vi "Autonomous Independent.vi"   [LabVIEW 2020]
doc: "This VI is called when autonomous begins, and will automatically be terminated when autonomous ends. You can carry out timed or sensor driven robot movement independently without needing to return to the caller."
uses:
  <vilib>/Rock Robotics/WPI/Utilities/WPI_GetSetVariantRefNum.vi
  <vilib>/Rock Robotics/Network Tables/NT Read String.vi
  <vilib>/Rock Robotics/Network Tables/NT Write Numeric Array.vi
panel:
  # "Be sure to right-click and choose Data Operations>>Make Current Value default if you want to save the array values with the VI"
  # "Click here to set max"
  # "Click here to set min"
types:
  T1 = typedef "WPI_JoystickDevRef.ctl" = cluster{"Device":T2}
  T2 = typedef "WPI_JoystickDeviceEnum.ctl" = enum16{"USB 0", "USB 1", "USB 2", "USB 3", "USB 4", "USB 5"}
  T3 = typedef "WPI_MotorControlDeviceRef.ctl" = cluster{"DeviceStatus":errorcluster, "Type":T4, "PWM":cluster{"PWM Channel":T5, "DeadBand":T6}, "CAN":cluster{"Device Number":u8, "SetOutput VI Ref":variant, "GetOutput VI Ref":variant, "Enable VI Ref":variant, "Disable VI Ref":variant, "Data":variant}, "Invert":bool, "DIO PWM":cluster{"PWM \"Enable\" Channel":T5, "DIOChannel":T7, "PWM Rate":dbl}}
  T4 = typedef "WPI_MotorControlType.ctl" = enum16{"PWM", "CAN", "DIO PWM"}
  T5 = typedef "FPGA_DIOPWMChannel.ctl" = enum8{"PWM 0", "PWM 1", "PWM 2", "PWM 3", "PWM 4", "PWM 5", "PWM 6", "PWM 7", "PWM 8", "PWM 9", "PWM MXP 0", "PWM MXP 1", "PWM MXP 2", "PWM MXP 3", "PWM MXP 4", "PWM MXP 5", "PWM MXP 6", "PWM MXP 7", "PWM MXP 8", "PWM MXP 9", "Invalid"}
  T6 = typedef "WPI_PWMDeadband.ctl" = cluster{"Name":string, "maxPositivePwm":i32, "minPositivePwm":i32, "centerPwm":i32, "maxNegativePwm":i32, "minNegativePwm":i32, "angularRange":u16}
  T7 = typedef "FPGA_DIOChannel.ctl" = enum8{"DIO 0", "DIO 1", "DIO 2", "DIO 3", "DIO 4", "DIO 5", "DIO 6", "DIO 7", "DIO 8", "DIO 9", "DIO MXP 0", "DIO MXP 1", "DIO MXP 2", "DIO MXP 3", "DIO MXP 4", "DIO MXP 5", "DIO MXP 6", "DIO MXP 7", "DIO MXP 8", "DIO MXP 9", "DIO MXP 10", "DIO MXP 11", "DIO MXP 12", "DIO MXP 13", "DIO MXP 14", "DIO MXP 15", "SPI Port CS1", "SPI Port CS2", "SPI Port CS3", "SPI Port MISO", "SPI Port MOSI", "Invalid"}
  T8 = typedef "WPI_RobotDriveDevRef.ctl" = cluster{"DevStatus":errorcluster, "Motors[]":T3[], "Square Inputs":bool, "Max Output":dbl}
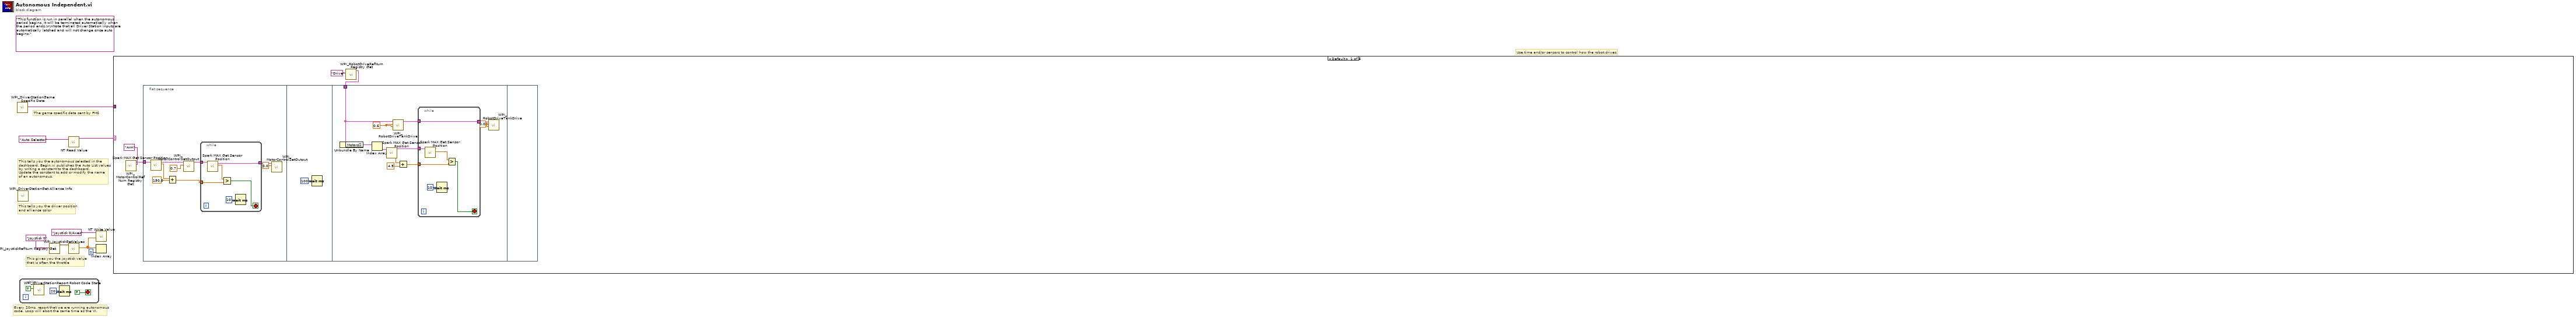
[diagram p0: block diagram]
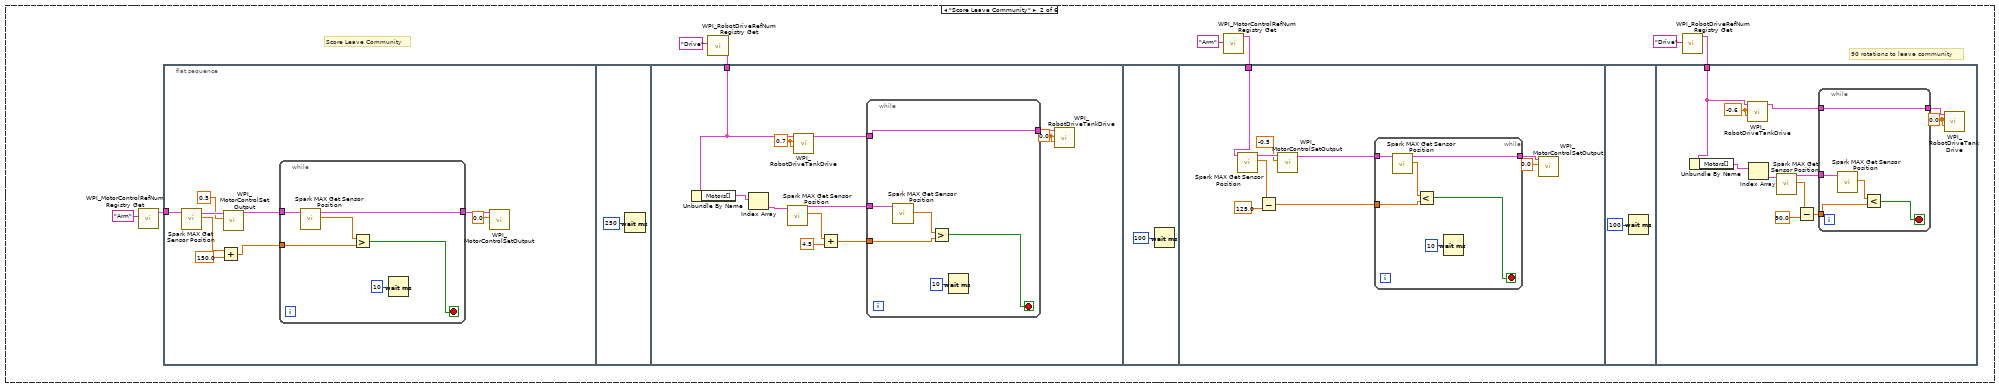
[diagram p2: hidden frame]
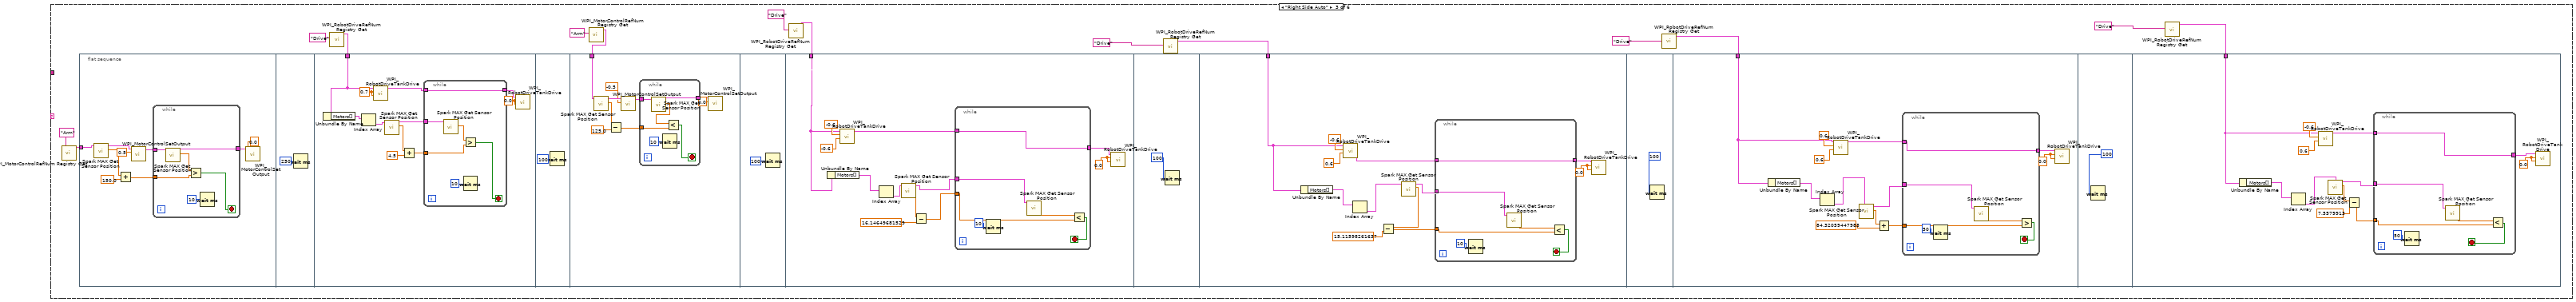
[diagram p3: hidden frame]
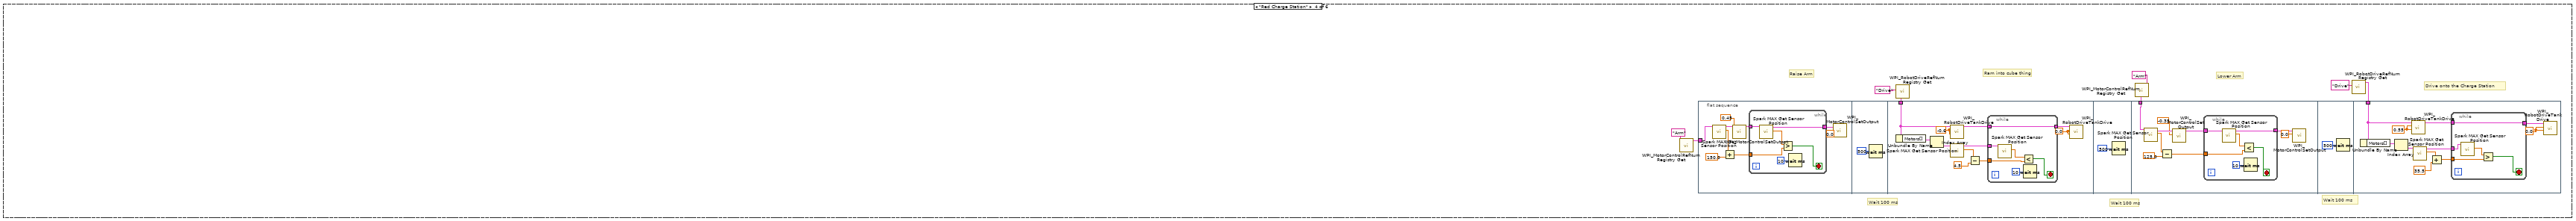
[diagram p4: hidden frame]
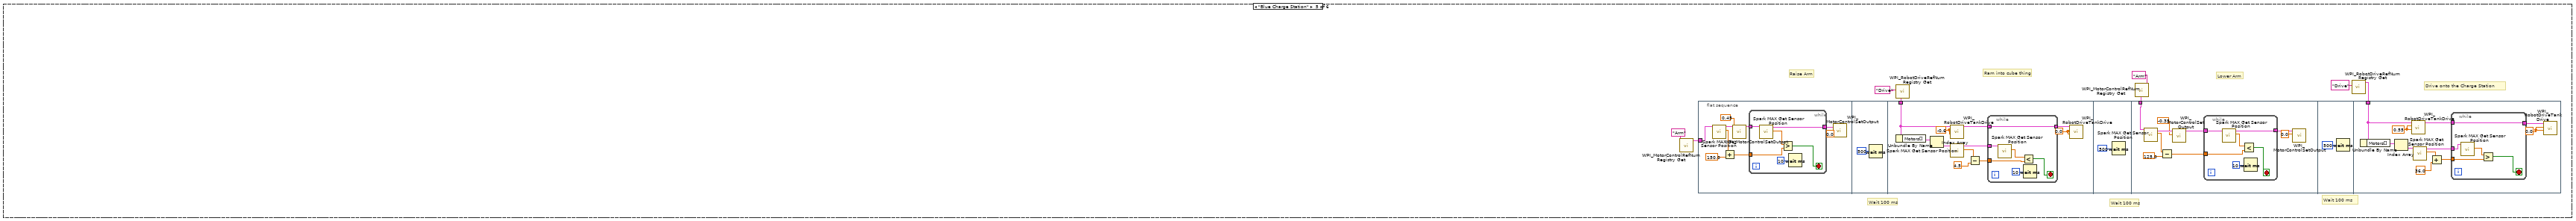
[diagram p5: hidden frame]
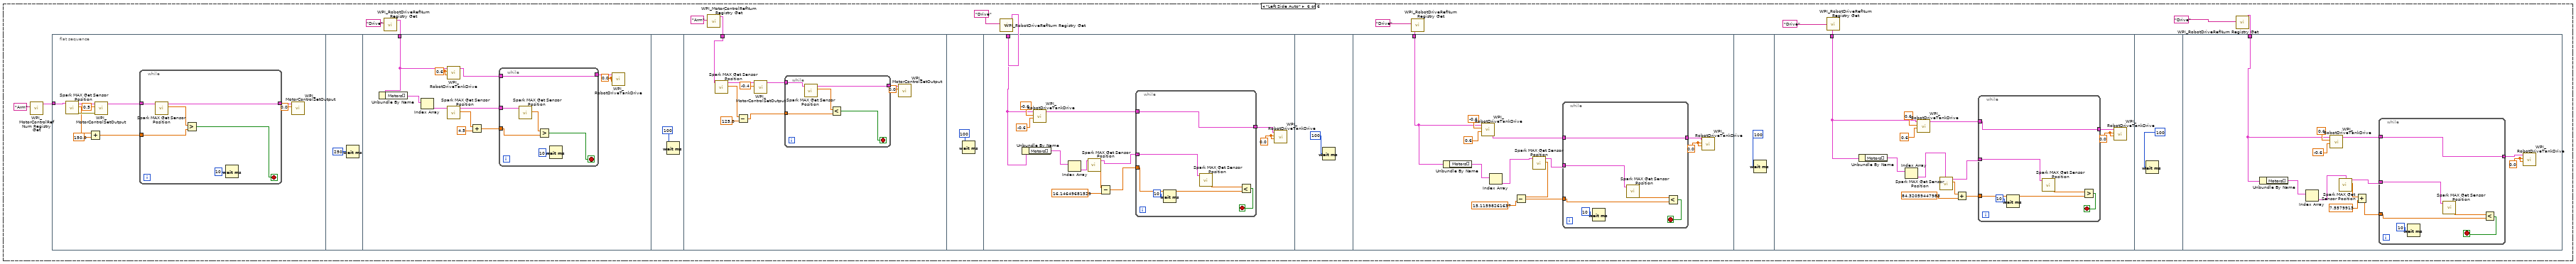
[diagram p6: hidden frame]
diagram:
  (unwired) "This function is run in parallel when the autonomous period begins. It will be terminated automatically when the period ends.\n\nNote that all Driver Station inputs are automatically latched and will not change once auto begins."
  # "The game specific data sent by FMS"
  # "This tells you the autonomous selected in the \ndashboard. Begin.vi publishes the Auto List values\nby writing a constant to the dashboard.\nUpdate the constant to add or modify the name\nof an autonomous."
  # "Every 20ms, report that we are running autonomous\ncode. Loop will abort the same time as the VI."
  # "This gives you the joystick value\nthat is often the throttle"
  # "Use time and/or sensors to control how the robot drives."
  # "This tells you the driver position\nand alliance color"
  n1 = call <vilib>:"WPI_DriverStationGame Specific Data.vi"() -> ("Game Specific Data"=w1:string)  [unwired: 11 in]
  n2 = call <vilib>:"WPI_DriverStationGet Alliance Info.vi"() -> ()  [unwired: 12 out]
  n3 = while {
    stop <- FALSE stop-if-true
    n4 = call <vilib>:"WPI_DriverStationReport Robot Code State.vi"("Autonomous"=TRUE) -> ()  [unwired: 10 in, 1 out]
    n5 = Wait (ms)(milliseconds to wait=u32 20) -> ()  [unwired: 1 out]
  }
  n6 = call <vilib>:"WPI_JoystickRefNum Registry Get.vi"("refnum name"="Joystick 0") -> ("JoystickDevRef"=w7:T1)  [unwired: 1 in, 9 out]
  n7 = call <vilib>:"WPI_JoystickGetValues.vi"("JoystickDevRef"=w7) -> ("Axes"=w3:dbl[])  [unwired: 6 in, 4 out]
  n8 = call-poly <vilib>:"NT Read Value.vi"("name"="Auto Selector" ("Name")) -> ("value"=w4:string)  [unwired: 8 in, 2 out]
  n9 = call-poly <vilib>:"NT Write Value.vi"("value"=w3, "name"="Joystick 0/Axes" ("Name")) -> ()  [unwired: 9 in, 1 out]
  n10 = Index Array(array=w3, index=2) -> ()  [unwired: 1 out]
  n11 = case shown="Default" w4 {
    tunnel: w1 -> [_ _ _ _ _ _]
    frame Default {
      n12 = call <vilib>:"WPI_MotorControlRefNum Registry Get.vi"("refnum name"="Arm") -> ("MotorControlDevRef"=w14:T3)  [unwired: 9 in, 1 out]
      n13 = flat-sequence {
        tunnel: w14 -> [w24]
        tunnel: w12 -> [w41]
        frame #0 {
          n14 = call <vilib>:"Spark MAX Get Sensor Position.vi"("MotorControlDevRef in"=w24) -> ("Sensor Position"=w23:dbl, "MotorControlDevRef out"=w21:T3)  [unwired: 7 in, 2 out]
          n15 = Add(x=w23, y=150.0) -> (x+y=w18:dbl)
          n16 = call <vilib>:"WPI_MotorControlSetOutput.vi"("Output"=0.7, "MotorControlDevRef"=w21) -> ("MotorControlDevRef"=w19:T3)  [unwired: 7 in, 2 out]
          n17 = while {
            tunnel: w19 -> [w30]
            tunnel: w18 -> [w28]
            tunnel: [w25] -> w17
            stop <- w27 stop-if-true
            n18 = call <vilib>:"Spark MAX Get Sensor Position.vi"("MotorControlDevRef in"=w30) -> ("Sensor Position"=w29:dbl, "MotorControlDevRef out"=w25:T3)  [unwired: 7 in, 2 out]
            n19 = Greater?(x=w29, y=w28) -> (0:w27:bool)
            n20 = Wait (ms)(milliseconds to wait=u32 10) -> ()  [unwired: 1 out]
          }
          n21 = call <vilib>:"WPI_MotorControlSetOutput.vi"("Output"=0.0, "MotorControlDevRef"=w17) -> ()  [unwired: 7 in, 3 out]
        }
        frame #1 {
          n22 = Wait (ms)(milliseconds to wait=u32 100) -> ()  [unwired: 1 out]
        }
        frame #2 {
          w32 = 0.0 ("Left axis value")
          w38 = 0.6 ("Left axis value")
          n23 = Unbundle By Name(w41) -> ("Motors[]"=w42:T3[])
          n24 = Index Array(array=w42) -> (element=w40:T3)  [unwired: 1 in]
          n25 = call <vilib>:"Spark MAX Get Sensor Position.vi"("MotorControlDevRef in"=w40) -> ("Sensor Position"=w39:dbl, "MotorControlDevRef out"=w36:T3)  [unwired: 7 in, 2 out]
          n26 = call <vilib>:"WPI_RobotDriveTankDrive.vi"("Right axis value"=w38, "Left axis value"=w38, "RobotDriveDevRef"=w41) -> ("RobotDriveDevRef"=w34:T8)  [unwired: 6 in, 2 out]
          n27 = Add(x=w39, y=4.5) -> (x+y=w35:dbl)
          n28 = while {
            tunnel: w36 -> [w48]
            tunnel: w35 -> [w47]
            tunnel: [w43] -> w33
            tunnel: w34 -> [w43]
            stop <- w45 stop-if-true
            n29 = call <vilib>:"Spark MAX Get Sensor Position.vi"("MotorControlDevRef in"=w48) -> ("Sensor Position"=w46:dbl)  [unwired: 7 in, 3 out]
            n30 = Wait (ms)(milliseconds to wait=u32 10) -> ()  [unwired: 1 out]
            n31 = Greater?(x=w46, y=w47) -> (0:w45:bool)
          }
          n32 = call <vilib>:"WPI_RobotDriveTankDrive.vi"("Right axis value"=w32, "Left axis value"=w32, "RobotDriveDevRef"=w33) -> ()  [unwired: 6 in, 3 out]
        }
        frame #3 {
        }
      }
      n33 = call <vilib>:"WPI_RobotDriveRefNum Registry Get.vi"("refnum name"="Drive") -> ("RobotDriveDevRef"=w12:T8)  [unwired: 9 in, 1 out]
    }
    frame "Score Leave Community" {
      # "90 rotations to leave community"
      # "Score Leave Community"
      n34 = call <vilib>:"WPI_MotorControlRefNum Registry Get.vi"("refnum name"="Arm") -> ("MotorControlDevRef"=w55:T3)  [unwired: 9 in, 1 out]
      n35 = flat-sequence {
        tunnel: w55 -> [w65]
        tunnel: w53 -> [w82]
        tunnel: w51 -> [w99]
        tunnel: w49 -> [w115]
        frame #0 {
          n36 = call <vilib>:"Spark MAX Get Sensor Position.vi"("MotorControlDevRef in"=w65) -> ("Sensor Position"=w63:dbl, "MotorControlDevRef out"=w64:T3)  [unwired: 7 in, 2 out]
          n37 = Add(x=w63, y=150.0) -> (x+y=w59:dbl)
          n38 = call <vilib>:"WPI_MotorControlSetOutput.vi"("Output"=0.5, "MotorControlDevRef"=w64) -> ("MotorControlDevRef"=w60:T3)  [unwired: 7 in, 2 out]
          n39 = while {
            tunnel: w60 -> [w71]
            tunnel: w59 -> [w69]
            tunnel: [w66] -> w58
            stop <- w68 stop-if-true
            n40 = call <vilib>:"Spark MAX Get Sensor Position.vi"("MotorControlDevRef in"=w71) -> ("Sensor Position"=w70:dbl, "MotorControlDevRef out"=w66:T3)  [unwired: 7 in, 2 out]
            n41 = Greater?(x=w70, y=w69) -> (0:w68:bool)
            n42 = Wait (ms)(milliseconds to wait=u32 10) -> ()  [unwired: 1 out]
          }
          n43 = call <vilib>:"WPI_MotorControlSetOutput.vi"("Output"=0.0, "MotorControlDevRef"=w58) -> ()  [unwired: 7 in, 3 out]
        }
        frame #1 {
          n44 = Wait (ms)(milliseconds to wait=u32 250) -> ()  [unwired: 1 out]
        }
        frame #2 {
          w73 = 0.0 ("Left axis value")
          w78 = 0.7 ("Left axis value")
          n45 = Unbundle By Name(w82) -> ("Motors[]"=w83:T3[])
          n46 = Index Array(array=w83) -> (element=w81:T3)  [unwired: 1 in]
          n47 = call <vilib>:"Spark MAX Get Sensor Position.vi"("MotorControlDevRef in"=w81) -> ("Sensor Position"=w80:dbl, "MotorControlDevRef out"=w77:T3)  [unwired: 7 in, 2 out]
          n48 = call <vilib>:"WPI_RobotDriveTankDrive.vi"("Right axis value"=w78, "Left axis value"=w78, "RobotDriveDevRef"=w82) -> ("RobotDriveDevRef"=w75:T8)  [unwired: 6 in, 2 out]
          n49 = Add(x=w80, y=4.5) -> (x+y=w76:dbl)
          n50 = while {
            tunnel: w77 -> [w89]
            tunnel: w76 -> [w87]
            tunnel: w75 -> [w84]
            tunnel: [w84] -> w74
            stop <- w86 stop-if-true
            n51 = call <vilib>:"Spark MAX Get Sensor Position.vi"("MotorControlDevRef in"=w89) -> ("Sensor Position"=w88:dbl)  [unwired: 7 in, 3 out]
            n52 = Greater?(x=w88, y=w87) -> (0:w86:bool)
            n53 = Wait (ms)(milliseconds to wait=u32 10) -> ()  [unwired: 1 out]
          }
          n54 = call <vilib>:"WPI_RobotDriveTankDrive.vi"("Right axis value"=w73, "Left axis value"=w73, "RobotDriveDevRef"=w74) -> ()  [unwired: 6 in, 3 out]
        }
        frame #3 {
          n55 = Wait (ms)(milliseconds to wait=u32 100) -> ()  [unwired: 1 out]
        }
        frame #4 {
          n56 = call <vilib>:"Spark MAX Get Sensor Position.vi"("MotorControlDevRef in"=w99) -> ("Sensor Position"=w96:dbl, "MotorControlDevRef out"=w98:T3)  [unwired: 7 in, 2 out]
          n57 = Subtract(x=w96, y=125.0) -> (x-y=w93:dbl)
          n58 = call <vilib>:"WPI_MotorControlSetOutput.vi"("Output"=-0.5, "MotorControlDevRef"=w98) -> ("MotorControlDevRef"=w94:T3)  [unwired: 7 in, 2 out]
          n59 = while {
            tunnel: w94 -> [w105]
            tunnel: w93 -> [w103]
            tunnel: [w100] -> w92
            stop <- w102 stop-if-true
            n60 = call <vilib>:"Spark MAX Get Sensor Position.vi"("MotorControlDevRef in"=w105) -> ("Sensor Position"=w104:dbl, "MotorControlDevRef out"=w100:T3)  [unwired: 7 in, 2 out]
            n61 = Less?(x=w104, y=w103) -> (x < y?=w102:bool)
            n62 = Wait (ms)(milliseconds to wait=u32 10) -> ()  [unwired: 1 out]
          }
          n63 = call <vilib>:"WPI_MotorControlSetOutput.vi"("Output"=0.0, "MotorControlDevRef"=w92) -> ()  [unwired: 7 in, 3 out]
        }
        frame #5 {
          n64 = Wait (ms)(milliseconds to wait=u32 100) -> ()  [unwired: 1 out]
        }
        frame #6 {
          w109 = 0.0 ("Left axis value")
          w116 = -0.6 ("Left axis value")
          n65 = Unbundle By Name(w115) -> ("Motors[]"=w117:T3[])
          n66 = call <vilib>:"WPI_RobotDriveTankDrive.vi"("Right axis value"=w116, "Left axis value"=w116, "RobotDriveDevRef"=w115) -> ("RobotDriveDevRef"=w108:T8)  [unwired: 6 in, 2 out]
          n67 = Index Array(array=w117) -> (element=w114:T3)  [unwired: 1 in]
          n68 = call <vilib>:"Spark MAX Get Sensor Position.vi"("MotorControlDevRef in"=w114) -> ("Sensor Position"=w113:dbl, "MotorControlDevRef out"=w111:T3)  [unwired: 7 in, 2 out]
          n69 = Subtract(x=w113, y=90.0) -> (x-y=w110:dbl)
          n70 = while {
            tunnel: w111 -> [w122]
            tunnel: w110 -> [w121]
            tunnel: [w118] -> w107
            tunnel: w108 -> [w118]
            stop <- w119 stop-if-true
            n71 = call <vilib>:"Spark MAX Get Sensor Position.vi"("MotorControlDevRef in"=w122) -> ("Sensor Position"=w120:dbl)  [unwired: 7 in, 3 out]
            n72 = Less?(x=w120, y=w121) -> (x < y?=w119:bool)
          }
          n73 = call <vilib>:"WPI_RobotDriveTankDrive.vi"("Right axis value"=w109, "Left axis value"=w109, "RobotDriveDevRef"=w107) -> ()  [unwired: 6 in, 3 out]
        }
      }
      n74 = call <vilib>:"WPI_RobotDriveRefNum Registry Get.vi"("refnum name"="Drive") -> ("RobotDriveDevRef"=w53:T8)  [unwired: 9 in, 1 out]
      n75 = call <vilib>:"WPI_MotorControlRefNum Registry Get.vi"("refnum name"="Arm") -> ("MotorControlDevRef"=w51:T3)  [unwired: 9 in, 1 out]
      n76 = call <vilib>:"WPI_RobotDriveRefNum Registry Get.vi"("refnum name"="Drive") -> ("RobotDriveDevRef"=w49:T8)  [unwired: 9 in, 1 out]
    }
    frame "Right Side Auto" {
      n77 = call <vilib>:"WPI_MotorControlRefNum Registry Get.vi"("refnum name"="Arm") -> ("MotorControlDevRef"=w127:T3)  [unwired: 9 in, 1 out]
      n78 = flat-sequence {
        tunnel: w127 -> [w145]
        tunnel: w125 -> [w162]
        tunnel: w123 -> [w179]
        tunnel: w135 -> [w193]
        tunnel: w133 -> [w210]
        tunnel: w131 -> [w227]
        tunnel: w129 -> [w244]
        frame #0 {
          n79 = call <vilib>:"Spark MAX Get Sensor Position.vi"("MotorControlDevRef in"=w145) -> ("Sensor Position"=w144:dbl, "MotorControlDevRef out"=w142:T3)  [unwired: 7 in, 2 out]
          n80 = Add(x=w144, y=150.0) -> (x+y=w137:dbl)
          n81 = call <vilib>:"WPI_MotorControlSetOutput.vi"("Output"=0.5, "MotorControlDevRef"=w142) -> ("MotorControlDevRef"=w140:T3)  [unwired: 7 in, 2 out]
          n82 = while {
            tunnel: w140 -> [w151]
            tunnel: [w150] -> w139
            tunnel: w137 -> [w148]
            stop <- w147 stop-if-true
            n83 = call <vilib>:"Spark MAX Get Sensor Position.vi"("MotorControlDevRef in"=w151) -> ("Sensor Position"=w149:dbl, "MotorControlDevRef out"=w150:T3)  [unwired: 7 in, 2 out]
            n84 = Greater?(x=w149, y=w148) -> (0:w147:bool)
            n85 = Wait (ms)(milliseconds to wait=u32 10) -> ()  [unwired: 1 out]
          }
          n86 = call <vilib>:"WPI_MotorControlSetOutput.vi"("Output"=0.0, "MotorControlDevRef"=w139) -> ()  [unwired: 7 in, 3 out]
        }
        frame #1 {
          n87 = Wait (ms)(milliseconds to wait=u32 250) -> ()  [unwired: 1 out]
        }
        frame #2 {
          w154 = 0.7 ("Left axis value")
          w153 = 0.0 ("Left axis value")
          n88 = Unbundle By Name(w162) -> ("Motors[]"=w163:T3[])
          n89 = Index Array(array=w163) -> (element=w161:T3)  [unwired: 1 in]
          n90 = call <vilib>:"WPI_RobotDriveTankDrive.vi"("Right axis value"=w154, "Left axis value"=w154, "RobotDriveDevRef"=w162) -> ("RobotDriveDevRef"=w155:T8)  [unwired: 6 in, 2 out]
          n91 = call <vilib>:"Spark MAX Get Sensor Position.vi"("MotorControlDevRef in"=w161) -> ("Sensor Position"=w159:dbl, "MotorControlDevRef out"=w158:T3)  [unwired: 7 in, 2 out]
          n92 = Add(x=w159, y=4.5) -> (x+y=w157:dbl)
          n93 = while {
            tunnel: w158 -> [w169]
            tunnel: w157 -> [w167]
            tunnel: w155 -> [w164]
            tunnel: [w164] -> w156
            stop <- w166 stop-if-true
            n94 = call <vilib>:"Spark MAX Get Sensor Position.vi"("MotorControlDevRef in"=w169) -> ("Sensor Position"=w168:dbl)  [unwired: 7 in, 3 out]
            n95 = Greater?(x=w168, y=w167) -> (0:w166:bool)
            n96 = Wait (ms)(milliseconds to wait=u32 10) -> ()  [unwired: 1 out]
          }
          n97 = call <vilib>:"WPI_RobotDriveTankDrive.vi"("Right axis value"=w153, "Left axis value"=w153, "RobotDriveDevRef"=w156) -> ()  [unwired: 6 in, 3 out]
        }
        frame #3 {
          n98 = Wait (ms)(milliseconds to wait=u32 100) -> ()  [unwired: 1 out]
        }
        frame #4 {
          n99 = call <vilib>:"Spark MAX Get Sensor Position.vi"("MotorControlDevRef in"=w179) -> ("Sensor Position"=w177:dbl, "MotorControlDevRef out"=w176:T3)  [unwired: 7 in, 2 out]
          n100 = Subtract(x=w177, y=125.0) -> (x-y=w173:dbl)
          n101 = call <vilib>:"WPI_MotorControlSetOutput.vi"("Output"=-0.5, "MotorControlDevRef"=w176) -> ("MotorControlDevRef"=w174:T3)  [unwired: 7 in, 2 out]
          n102 = while {
            tunnel: w174 -> [w185]
            tunnel: w173 -> [w184]
            tunnel: [w180] -> w172
            stop <- w182 stop-if-true
            n103 = call <vilib>:"Spark MAX Get Sensor Position.vi"("MotorControlDevRef in"=w185) -> ("Sensor Position"=w183:dbl, "MotorControlDevRef out"=w180:T3)  [unwired: 7 in, 2 out]
            n104 = Wait (ms)(milliseconds to wait=u32 10) -> ()  [unwired: 1 out]
            n105 = Less?(x=w183, y=w184) -> (x < y?=w182:bool)
          }
          n106 = call <vilib>:"WPI_MotorControlSetOutput.vi"("Output"=0.0, "MotorControlDevRef"=w172) -> ()  [unwired: 7 in, 3 out]
        }
        frame #5 {
          n107 = Wait (ms)(milliseconds to wait=u32 100) -> ()  [unwired: 1 out]
        }
        frame #6 {
          w196 = 0.0
          n108 = Unbundle By Name(w193) -> ("Motors[]"=w198:T3[])
          n109 = call <vilib>:"WPI_RobotDriveTankDrive.vi"("Right axis value"=-0.6, "Left axis value"=-0.6, "RobotDriveDevRef"=w193) -> ("RobotDriveDevRef"=w192:T8)  [unwired: 6 in, 2 out]
          n110 = Index Array(array=w198) -> (element=w191:T3)  [unwired: 1 in]
          n111 = call <vilib>:"Spark MAX Get Sensor Position.vi"("MotorControlDevRef in"=w191) -> ("Sensor Position"=w189:dbl, "MotorControlDevRef out"=w190:T3)  [unwired: 7 in, 2 out]
          n112 = Subtract(x=w189, y=16.14649681529) -> (x-y=w188:dbl)
          n113 = while {
            tunnel: w190 -> [w202]
            tunnel: [w200] -> w197
            tunnel: w192 -> [w200]
            tunnel: w188 -> [w199]
            stop <- w203 stop-if-true
            n114 = Wait (ms)(milliseconds to wait=10) -> ()  [unwired: 1 out]
            n115 = call <vilib>:"Spark MAX Get Sensor Position.vi"("MotorControlDevRef in"=w202) -> ("Sensor Position"=w204:dbl)  [unwired: 7 in, 3 out]
            n116 = Less?(x=w204, y=w199) -> (x < y?=w203:bool)
          }
          n117 = call <vilib>:"WPI_RobotDriveTankDrive.vi"("Right axis value"=w196, "Left axis value"=w196, "RobotDriveDevRef"=w197) -> ()  [unwired: 6 in, 3 out]
        }
        frame #7 {
          n118 = Wait (ms)(milliseconds to wait=100) -> ()  [unwired: 1 out]
        }
        frame #8 {
          w214 = 0.0
          n119 = Unbundle By Name(w210) -> ("Motors[]"=w215:T3[])
          n120 = call <vilib>:"WPI_RobotDriveTankDrive.vi"("Right axis value"=0.6, "Left axis value"=-0.6, "RobotDriveDevRef"=w210) -> ("RobotDriveDevRef"=w209:T8)  [unwired: 6 in, 2 out]
          n121 = Index Array(array=w215) -> (element=w217:T3)  [unwired: 1 in]
          n122 = call <vilib>:"Spark MAX Get Sensor Position.vi"("MotorControlDevRef in"=w217) -> ("Sensor Position"=w208:dbl, "MotorControlDevRef out"=w216:T3)  [unwired: 7 in, 2 out]
          n123 = Subtract(x=w208, y=15.11598261637) -> (x-y=w206:dbl)
          n124 = while {
            tunnel: w216 -> [w221]
            tunnel: [w219] -> w213
            tunnel: w209 -> [w219]
            tunnel: w206 -> [w218]
            stop <- w222 stop-if-true
            n125 = Wait (ms)(milliseconds to wait=10) -> ()  [unwired: 1 out]
            n126 = call <vilib>:"Spark MAX Get Sensor Position.vi"("MotorControlDevRef in"=w221) -> ("Sensor Position"=w223:dbl)  [unwired: 7 in, 3 out]
            n127 = Less?(x=w223, y=w218) -> (x < y?=w222:bool)
          }
          n128 = call <vilib>:"WPI_RobotDriveTankDrive.vi"("Right axis value"=w214, "Left axis value"=w214, "RobotDriveDevRef"=w213) -> ()  [unwired: 6 in, 3 out]
        }
        frame #9 {
          n129 = Wait (ms)(milliseconds to wait=100) -> ()  [unwired: 1 out]
        }
        frame #10 {
          w233 = 0.0
          n130 = Unbundle By Name(w227) -> ("Motors[]"=w234:T3[])
          n131 = Index Array(array=w234) -> (element=w236:T3)  [unwired: 1 in]
          n132 = call <vilib>:"WPI_RobotDriveTankDrive.vi"("Right axis value"=0.6, "Left axis value"=0.6, "RobotDriveDevRef"=w227) -> ("RobotDriveDevRef"=w226:T8)  [unwired: 6 in, 2 out]
          n133 = call <vilib>:"Spark MAX Get Sensor Position.vi"("MotorControlDevRef in"=w236) -> ("Sensor Position"=w231:dbl, "MotorControlDevRef out"=w235:T3)  [unwired: 7 in, 2 out]
          n134 = Add(x=w231, y=84.32059447983 ("Position")) -> (x+y=w225:dbl)
          n135 = while {
            tunnel: w235 -> [w240]
            tunnel: [w238] -> w232
            tunnel: w226 -> [w238]
            tunnel: w225 -> [w237]
            stop <- w241 stop-if-true
            n136 = Wait (ms)(milliseconds to wait=50) -> ()  [unwired: 1 out]
            n137 = call <vilib>:"Spark MAX Get Sensor Position.vi"("MotorControlDevRef in"=w240) -> ("Sensor Position"=w242:dbl)  [unwired: 7 in, 3 out]
            n138 = Greater?(x=w242, y=w237) -> (0:w241:bool)
          }
          n139 = call <vilib>:"WPI_RobotDriveTankDrive.vi"("Right axis value"=w233, "Left axis value"=w233, "RobotDriveDevRef"=w232) -> ()  [unwired: 6 in, 3 out]
        }
        frame #11 {
          n140 = Wait (ms)(milliseconds to wait=100) -> ()  [unwired: 1 out]
        }
        frame #12 {
          w252 = 0.0
          n141 = Unbundle By Name(w244) -> ("Motors[]"=w253:T3[])
          n142 = Index Array(array=w253) -> (element=w255:T3)  [unwired: 1 in]
          n143 = call <vilib>:"WPI_RobotDriveTankDrive.vi"("Right axis value"=0.6, "Left axis value"=-0.6, "RobotDriveDevRef"=w244) -> ("RobotDriveDevRef"=w245:T8)  [unwired: 6 in, 2 out]
          n144 = call <vilib>:"Spark MAX Get Sensor Position.vi"("MotorControlDevRef in"=w255) -> ("Sensor Position"=w250:dbl, "MotorControlDevRef out"=w254:T3)  [unwired: 7 in, 2 out]
          n145 = Subtract(x=w250, y=7.5579913 ("Position")) -> (x-y=w248:dbl)
          n146 = while {
            tunnel: w254 -> [w259]
            tunnel: [w256] -> w251
            tunnel: w248 -> [w257]
            tunnel: w245 -> [w256]
            stop <- w260 stop-if-true
            n147 = Wait (ms)(milliseconds to wait=50) -> ()  [unwired: 1 out]
            n148 = call <vilib>:"Spark MAX Get Sensor Position.vi"("MotorControlDevRef in"=w259) -> ("Sensor Position"=w261:dbl)  [unwired: 7 in, 3 out]
            n149 = Less?(x=w261, y=w257) -> (x < y?=w260:bool)
          }
          n150 = call <vilib>:"WPI_RobotDriveTankDrive.vi"("Right axis value"=w252, "Left axis value"=w252, "RobotDriveDevRef"=w251) -> ()  [unwired: 6 in, 3 out]
        }
      }
      n151 = call <vilib>:"WPI_RobotDriveRefNum Registry Get.vi"("refnum name"="Drive") -> ("RobotDriveDevRef"=w125:T8)  [unwired: 9 in, 1 out]
      n152 = call <vilib>:"WPI_MotorControlRefNum Registry Get.vi"("refnum name"="Arm") -> ("MotorControlDevRef"=w123:T3)  [unwired: 9 in, 1 out]
      n153 = call <vilib>:"WPI_RobotDriveRefNum Registry Get.vi"("refnum name"="Drive") -> ("RobotDriveDevRef"=w135:T8)  [unwired: 9 in, 1 out]
      n154 = call <vilib>:"WPI_RobotDriveRefNum Registry Get.vi"("refnum name"="Drive") -> ("RobotDriveDevRef"=w133:T8)  [unwired: 9 in, 1 out]
      n155 = call <vilib>:"WPI_RobotDriveRefNum Registry Get.vi"("refnum name"="Drive") -> ("RobotDriveDevRef"=w131:T8)  [unwired: 9 in, 1 out]
      n156 = call <vilib>:"WPI_RobotDriveRefNum Registry Get.vi"("refnum name"="Drive") -> ("RobotDriveDevRef"=w129:T8)  [unwired: 9 in, 1 out]
    }
    frame "Red Charge Station" {
      # "Wait 100 ms"
      # "Drive onto the Charge Station"
      # "Wait 100 ms"
      # "Wait 100 ms"
      # "Lower Arm"
      # "Ram into cube thing"
      # "Raise Arm"
      n157 = call <vilib>:"WPI_MotorControlRefNum Registry Get.vi"("refnum name"="Arm") -> ("MotorControlDevRef"=w268:T3)  [unwired: 9 in, 1 out]
      n158 = flat-sequence {
        tunnel: w268 -> [w277]
        tunnel: w266 -> [w296]
        tunnel: w264 -> [w312]
        tunnel: w263 -> [w330]
        frame #0 {
          n159 = call <vilib>:"Spark MAX Get Sensor Position.vi"("MotorControlDevRef in"=w277) -> ("Sensor Position"=w273:dbl, "MotorControlDevRef out"=w275:T3)  [unwired: 7 in, 2 out]
          n160 = Add(x=w273, y=150.0) -> (x+y=w270:dbl)
          n161 = call <vilib>:"WPI_MotorControlSetOutput.vi"("Output"=0.45, "MotorControlDevRef"=w275) -> ("MotorControlDevRef"=w276:T3)  [unwired: 7 in, 2 out]
          n162 = while {
            tunnel: w276 -> [w284]
            tunnel: [w282] -> w271
            tunnel: w270 -> [w279]
            stop <- w281 stop-if-true
            n163 = call <vilib>:"Spark MAX Get Sensor Position.vi"("MotorControlDevRef in"=w284) -> ("Sensor Position"=w280:dbl, "MotorControlDevRef out"=w282:T3)  [unwired: 7 in, 2 out]
            n164 = Greater?(x=w280, y=w279) -> (0:w281:bool)
            n165 = Wait (ms)(milliseconds to wait=u32 10) -> ()  [unwired: 1 out]
          }
          n166 = call <vilib>:"WPI_MotorControlSetOutput.vi"("Output"=0.0, "MotorControlDevRef"=w271) -> ()  [unwired: 7 in, 3 out]
        }
        frame #1 {
          n167 = Wait (ms)(milliseconds to wait=u32 500) -> ()  [unwired: 1 out]
        }
        frame #2 {
          w286 = -0.6 ("Left axis value")
          w287 = 0.0 ("Left axis value")
          n168 = Unbundle By Name(w296) -> ("Motors[]"=w295:T3[])
          n169 = Index Array(array=w295) -> (element=w294:T3)  [unwired: 1 in]
          n170 = call <vilib>:"WPI_RobotDriveTankDrive.vi"("Right axis value"=w286, "Left axis value"=w286, "RobotDriveDevRef"=w296) -> ("RobotDriveDevRef"=w291:T8)  [unwired: 6 in, 2 out]
          n171 = call <vilib>:"Spark MAX Get Sensor Position.vi"("MotorControlDevRef in"=w294) -> ("Sensor Position"=w293:dbl, "MotorControlDevRef out"=w290:T3)  [unwired: 7 in, 2 out]
          n172 = Subtract(x=w293, y=4.5) -> (x-y=w289:dbl)
          n173 = while {
            tunnel: [w302] -> w288
            tunnel: w291 -> [w302]
            tunnel: w290 -> [w301]
            tunnel: w289 -> [w300]
            stop <- w298 stop-if-true
            n174 = call <vilib>:"Spark MAX Get Sensor Position.vi"("MotorControlDevRef in"=w301) -> ("Sensor Position"=w299:dbl)  [unwired: 7 in, 3 out]
            n175 = Less?(x=w299, y=w300) -> (x < y?=w298:bool)
            n176 = Wait (ms)(milliseconds to wait=u32 10) -> ()  [unwired: 1 out]
          }
          n177 = call <vilib>:"WPI_RobotDriveTankDrive.vi"("Right axis value"=w287, "Left axis value"=w287, "RobotDriveDevRef"=w288) -> ()  [unwired: 6 in, 3 out]
        }
        frame #3 {
          n178 = Wait (ms)(milliseconds to wait=u32 500) -> ()  [unwired: 1 out]
        }
        frame #4 {
          n179 = call <vilib>:"Spark MAX Get Sensor Position.vi"("MotorControlDevRef in"=w312) -> ("Sensor Position"=w309:dbl, "MotorControlDevRef out"=w311:T3)  [unwired: 7 in, 2 out]
          n180 = Subtract(x=w309, y=125.0) -> (x-y=w307:dbl)
          n181 = call <vilib>:"WPI_MotorControlSetOutput.vi"("Output"=-0.35, "MotorControlDevRef"=w311) -> ("MotorControlDevRef"=w306:T3)  [unwired: 7 in, 2 out]
          n182 = while {
            tunnel: w307 -> [w317]
            tunnel: w306 -> [w315]
            tunnel: [w313] -> w305
            stop <- w314 stop-if-true
            n183 = call <vilib>:"Spark MAX Get Sensor Position.vi"("MotorControlDevRef in"=w315) -> ("Sensor Position"=w316:dbl, "MotorControlDevRef out"=w313:T3)  [unwired: 7 in, 2 out]
            n184 = Less?(x=w316, y=w317) -> (x < y?=w314:bool)
            n185 = Wait (ms)(milliseconds to wait=u32 10) -> ()  [unwired: 1 out]
          }
          n186 = call <vilib>:"WPI_MotorControlSetOutput.vi"("Output"=0.0, "MotorControlDevRef"=w305) -> ()  [unwired: 7 in, 3 out]
        }
        frame #5 {
          n187 = Wait (ms)(milliseconds to wait=u32 500) -> ()  [unwired: 1 out]
        }
        frame #6 {
          w322 = 0.0 ("Right axis value")
          w328 = 0.55 ("Left axis value")
          n188 = Unbundle By Name(w330) -> ("Motors[]"=w329:T3[])
          n189 = Index Array(array=w329) -> (element=w327:T3)  [unwired: 1 in]
          n190 = call <vilib>:"WPI_RobotDriveTankDrive.vi"("Right axis value"=w328, "Left axis value"=w328, "RobotDriveDevRef"=w330) -> ("RobotDriveDevRef"=w321:T8)  [unwired: 6 in, 2 out]
          n191 = call <vilib>:"Spark MAX Get Sensor Position.vi"("MotorControlDevRef in"=w327) -> ("Sensor Position"=w326:dbl, "MotorControlDevRef out"=w324:T3)  [unwired: 7 in, 2 out]
          n192 = Add(x=w326, y=35.5) -> (x+y=w323:dbl)
          n193 = while {
            tunnel: w324 -> [w335]
            tunnel: w323 -> [w334]
            tunnel: [w331] -> w320
            tunnel: w321 -> [w331]
            stop <- w332 stop-if-true
            n194 = call <vilib>:"Spark MAX Get Sensor Position.vi"("MotorControlDevRef in"=w335) -> ("Sensor Position"=w333:dbl)  [unwired: 7 in, 3 out]
            n195 = Greater?(x=w333, y=w334) -> (0:w332:bool)
          }
          n196 = call <vilib>:"WPI_RobotDriveTankDrive.vi"("Right axis value"=w322, "Left axis value"=w322, "RobotDriveDevRef"=w320) -> ()  [unwired: 6 in, 3 out]
        }
      }
      n197 = call <vilib>:"WPI_RobotDriveRefNum Registry Get.vi"("refnum name"="Drive") -> ("RobotDriveDevRef"=w266:T8)  [unwired: 9 in, 1 out]
      n198 = call <vilib>:"WPI_MotorControlRefNum Registry Get.vi"("refnum name"="Arm") -> ("MotorControlDevRef"=w264:T3)  [unwired: 9 in, 1 out]
      n199 = call <vilib>:"WPI_RobotDriveRefNum Registry Get.vi"("refnum name"="Drive") -> ("RobotDriveDevRef"=w263:T8)  [unwired: 9 in, 1 out]
    }
    frame "Blue Charge Station" {
      # "Wait 100 ms"
      # "Drive onto the Charge Station"
      # "Wait 100 ms"
      # "Wait 100 ms"
      # "Lower Arm"
      # "Ram into cube thing"
      # "Raise Arm"
      n200 = call <vilib>:"WPI_MotorControlRefNum Registry Get.vi"("refnum name"="Arm") -> ("MotorControlDevRef"=w342:T3)  [unwired: 9 in, 1 out]
      n201 = flat-sequence {
        tunnel: w342 -> [w351]
        tunnel: w340 -> [w370]
        tunnel: w338 -> [w386]
        tunnel: w337 -> [w404]
        frame #0 {
          n202 = call <vilib>:"Spark MAX Get Sensor Position.vi"("MotorControlDevRef in"=w351) -> ("Sensor Position"=w347:dbl, "MotorControlDevRef out"=w349:T3)  [unwired: 7 in, 2 out]
          n203 = Add(x=w347, y=150.0) -> (x+y=w344:dbl)
          n204 = call <vilib>:"WPI_MotorControlSetOutput.vi"("Output"=0.45, "MotorControlDevRef"=w349) -> ("MotorControlDevRef"=w350:T3)  [unwired: 7 in, 2 out]
          n205 = while {
            tunnel: w350 -> [w358]
            tunnel: [w356] -> w345
            tunnel: w344 -> [w353]
            stop <- w355 stop-if-true
            n206 = call <vilib>:"Spark MAX Get Sensor Position.vi"("MotorControlDevRef in"=w358) -> ("Sensor Position"=w354:dbl, "MotorControlDevRef out"=w356:T3)  [unwired: 7 in, 2 out]
            n207 = Greater?(x=w354, y=w353) -> (0:w355:bool)
            n208 = Wait (ms)(milliseconds to wait=u32 10) -> ()  [unwired: 1 out]
          }
          n209 = call <vilib>:"WPI_MotorControlSetOutput.vi"("Output"=0.0, "MotorControlDevRef"=w345) -> ()  [unwired: 7 in, 3 out]
        }
        frame #1 {
          n210 = Wait (ms)(milliseconds to wait=u32 500) -> ()  [unwired: 1 out]
        }
        frame #2 {
          w360 = -0.6 ("Left axis value")
          w361 = 0.0 ("Left axis value")
          n211 = Unbundle By Name(w370) -> ("Motors[]"=w369:T3[])
          n212 = Index Array(array=w369) -> (element=w368:T3)  [unwired: 1 in]
          n213 = call <vilib>:"WPI_RobotDriveTankDrive.vi"("Right axis value"=w360, "Left axis value"=w360, "RobotDriveDevRef"=w370) -> ("RobotDriveDevRef"=w365:T8)  [unwired: 6 in, 2 out]
          n214 = call <vilib>:"Spark MAX Get Sensor Position.vi"("MotorControlDevRef in"=w368) -> ("Sensor Position"=w367:dbl, "MotorControlDevRef out"=w364:T3)  [unwired: 7 in, 2 out]
          n215 = Subtract(x=w367, y=4.5) -> (x-y=w363:dbl)
          n216 = while {
            tunnel: [w376] -> w362
            tunnel: w365 -> [w376]
            tunnel: w364 -> [w375]
            tunnel: w363 -> [w374]
            stop <- w372 stop-if-true
            n217 = call <vilib>:"Spark MAX Get Sensor Position.vi"("MotorControlDevRef in"=w375) -> ("Sensor Position"=w373:dbl)  [unwired: 7 in, 3 out]
            n218 = Less?(x=w373, y=w374) -> (x < y?=w372:bool)
            n219 = Wait (ms)(milliseconds to wait=u32 10) -> ()  [unwired: 1 out]
          }
          n220 = call <vilib>:"WPI_RobotDriveTankDrive.vi"("Right axis value"=w361, "Left axis value"=w361, "RobotDriveDevRef"=w362) -> ()  [unwired: 6 in, 3 out]
        }
        frame #3 {
          n221 = Wait (ms)(milliseconds to wait=u32 500) -> ()  [unwired: 1 out]
        }
        frame #4 {
          n222 = call <vilib>:"Spark MAX Get Sensor Position.vi"("MotorControlDevRef in"=w386) -> ("Sensor Position"=w383:dbl, "MotorControlDevRef out"=w385:T3)  [unwired: 7 in, 2 out]
          n223 = Subtract(x=w383, y=125.0) -> (x-y=w381:dbl)
          n224 = call <vilib>:"WPI_MotorControlSetOutput.vi"("Output"=-0.35, "MotorControlDevRef"=w385) -> ("MotorControlDevRef"=w380:T3)  [unwired: 7 in, 2 out]
          n225 = while {
            tunnel: w381 -> [w391]
            tunnel: w380 -> [w389]
            tunnel: [w387] -> w379
            stop <- w388 stop-if-true
            n226 = call <vilib>:"Spark MAX Get Sensor Position.vi"("MotorControlDevRef in"=w389) -> ("Sensor Position"=w390:dbl, "MotorControlDevRef out"=w387:T3)  [unwired: 7 in, 2 out]
            n227 = Less?(x=w390, y=w391) -> (x < y?=w388:bool)
            n228 = Wait (ms)(milliseconds to wait=u32 10) -> ()  [unwired: 1 out]
          }
          n229 = call <vilib>:"WPI_MotorControlSetOutput.vi"("Output"=0.0, "MotorControlDevRef"=w379) -> ()  [unwired: 7 in, 3 out]
        }
        frame #5 {
          n230 = Wait (ms)(milliseconds to wait=u32 500) -> ()  [unwired: 1 out]
        }
        frame #6 {
          w396 = 0.0 ("Right axis value")
          w402 = 0.55 ("Left axis value")
          n231 = Unbundle By Name(w404) -> ("Motors[]"=w403:T3[])
          n232 = Index Array(array=w403) -> (element=w401:T3)  [unwired: 1 in]
          n233 = call <vilib>:"WPI_RobotDriveTankDrive.vi"("Right axis value"=w402, "Left axis value"=w402, "RobotDriveDevRef"=w404) -> ("RobotDriveDevRef"=w395:T8)  [unwired: 6 in, 2 out]
          n234 = call <vilib>:"Spark MAX Get Sensor Position.vi"("MotorControlDevRef in"=w401) -> ("Sensor Position"=w400:dbl, "MotorControlDevRef out"=w398:T3)  [unwired: 7 in, 2 out]
          n235 = Add(x=w400, y=36.0) -> (x+y=w397:dbl)
          n236 = while {
            tunnel: w398 -> [w409]
            tunnel: w397 -> [w408]
            tunnel: [w405] -> w394
            tunnel: w395 -> [w405]
            stop <- w406 stop-if-true
            n237 = call <vilib>:"Spark MAX Get Sensor Position.vi"("MotorControlDevRef in"=w409) -> ("Sensor Position"=w407:dbl)  [unwired: 7 in, 3 out]
            n238 = Greater?(x=w407, y=w408) -> (0:w406:bool)
          }
          n239 = call <vilib>:"WPI_RobotDriveTankDrive.vi"("Right axis value"=w396, "Left axis value"=w396, "RobotDriveDevRef"=w394) -> ()  [unwired: 6 in, 3 out]
        }
      }
      n240 = call <vilib>:"WPI_RobotDriveRefNum Registry Get.vi"("refnum name"="Drive") -> ("RobotDriveDevRef"=w340:T8)  [unwired: 9 in, 1 out]
      n241 = call <vilib>:"WPI_MotorControlRefNum Registry Get.vi"("refnum name"="Arm") -> ("MotorControlDevRef"=w338:T3)  [unwired: 9 in, 1 out]
      n242 = call <vilib>:"WPI_RobotDriveRefNum Registry Get.vi"("refnum name"="Drive") -> ("RobotDriveDevRef"=w337:T8)  [unwired: 9 in, 1 out]
    }
    frame "Left Side Auto" {
      n243 = call <vilib>:"WPI_MotorControlRefNum Registry Get.vi"("refnum name"="Arm") -> ("MotorControlDevRef"=w414:T3)  [unwired: 9 in, 1 out]
      n244 = flat-sequence {
        tunnel: w414 -> [w433]
        tunnel: w412 -> [w450]
        tunnel: w410 -> [w467]
        tunnel: w422 -> [w480]
        tunnel: w420 -> [w497]
        tunnel: w418 -> [w514]
        tunnel: w416 -> [w531]
        frame #0 {
          n245 = call <vilib>:"Spark MAX Get Sensor Position.vi"("MotorControlDevRef in"=w433) -> ("error out"=w431:errorcluster, "Sensor Position"=w429:dbl, "MotorControlDevRef out"=w432:T3)  [unwired: 7 in, 1 out]
          n246 = Add(x=w429, y=150.0) -> (x+y=w426:dbl)
          n247 = call <vilib>:"WPI_MotorControlSetOutput.vi"("error in (no error)"=w431, "Output"=0.5, "MotorControlDevRef"=w432) -> ("MotorControlDevRef"=w427:T3)  [unwired: 6 in, 2 out]
          n248 = while {
            tunnel: w427 -> [w439]
            tunnel: w426 -> [w437]
            tunnel: [w434] -> w425
            stop <- w436 stop-if-true
            n249 = call <vilib>:"Spark MAX Get Sensor Position.vi"("MotorControlDevRef in"=w439) -> ("Sensor Position"=w438:dbl, "MotorControlDevRef out"=w434:T3)  [unwired: 7 in, 2 out]
            n250 = Greater?(x=w438, y=w437) -> (0:w436:bool)
            n251 = Wait (ms)(milliseconds to wait=u32 10) -> ()  [unwired: 1 out]
          }
          n252 = call <vilib>:"WPI_MotorControlSetOutput.vi"("Output"=0.0, "MotorControlDevRef"=w425) -> ()  [unwired: 7 in, 3 out]
        }
        frame #1 {
          n253 = Wait (ms)(milliseconds to wait=u32 250) -> ()  [unwired: 1 out]
        }
        frame #2 {
          w441 = 0.0 ("Left axis value")
          w446 = 0.6 ("Left axis value")
          n254 = Unbundle By Name(w450) -> ("Motors[]"=w451:T3[])
          n255 = Index Array(array=w451) -> (element=w449:T3)  [unwired: 1 in]
          n256 = call <vilib>:"Spark MAX Get Sensor Position.vi"("MotorControlDevRef in"=w449) -> ("Sensor Position"=w448:dbl, "MotorControlDevRef out"=w444:T3)  [unwired: 7 in, 2 out]
          n257 = call <vilib>:"WPI_RobotDriveTankDrive.vi"("Right axis value"=w446, "Left axis value"=w446, "RobotDriveDevRef"=w450) -> ("RobotDriveDevRef"=w443:T8)  [unwired: 6 in, 2 out]
          n258 = Add(x=w448, y=4.5) -> (x+y=w445:dbl)
          n259 = while {
            tunnel: w445 -> [w455]
            tunnel: w444 -> [w454]
            tunnel: [w452] -> w442
            tunnel: w443 -> [w452]
            stop <- w453 stop-if-true
            n260 = call <vilib>:"Spark MAX Get Sensor Position.vi"("MotorControlDevRef in"=w454) -> ("Sensor Position"=w456:dbl)  [unwired: 7 in, 3 out]
            n261 = Greater?(x=w456, y=w455) -> (0:w453:bool)
            n262 = Wait (ms)(milliseconds to wait=u32 10) -> ()  [unwired: 1 out]
          }
          n263 = call <vilib>:"WPI_RobotDriveTankDrive.vi"("Right axis value"=w441, "Left axis value"=w441, "RobotDriveDevRef"=w442) -> ()  [unwired: 6 in, 3 out]
        }
        frame #3 {
          n264 = Wait (ms)(milliseconds to wait=u32 100) -> ()  [unwired: 1 out]
        }
        frame #4 {
          n265 = call <vilib>:"Spark MAX Get Sensor Position.vi"("MotorControlDevRef in"=w467) -> ("Sensor Position"=w466:dbl, "MotorControlDevRef out"=w464:T3)  [unwired: 7 in, 2 out]
          n266 = Subtract(x=w466, y=125.0) -> (x-y=w461:dbl)
          n267 = call <vilib>:"WPI_MotorControlSetOutput.vi"("Output"=-0.4, "MotorControlDevRef"=w464) -> ("MotorControlDevRef"=w462:T3)  [unwired: 7 in, 2 out]
          n268 = while {
            tunnel: w462 -> [w472]
            tunnel: w461 -> [w470]
            tunnel: [w468] -> w460
            stop <- w469 stop-if-true
            n269 = call <vilib>:"Spark MAX Get Sensor Position.vi"("MotorControlDevRef in"=w472) -> ("Sensor Position"=w471:dbl, "MotorControlDevRef out"=w468:T3)  [unwired: 7 in, 2 out]
            n270 = Less?(x=w471, y=w470) -> (x < y?=w469:bool)
          }
          n271 = call <vilib>:"WPI_MotorControlSetOutput.vi"("Output"=0.0, "MotorControlDevRef"=w460) -> ()  [unwired: 7 in, 3 out]
        }
        frame #5 {
          n272 = Wait (ms)(milliseconds to wait=u32 100) -> ()  [unwired: 1 out]
        }
        frame #6 {
          w483 = 0.0
          n273 = Unbundle By Name(w480) -> ("Motors[]"=w485:T3[])
          n274 = call <vilib>:"WPI_RobotDriveTankDrive.vi"("Right axis value"=-0.6, "Left axis value"=-0.6, "RobotDriveDevRef"=w480) -> ("RobotDriveDevRef"=w479:T8)  [unwired: 6 in, 2 out]
          n275 = Index Array(array=w485) -> (element=w478:T3)  [unwired: 1 in]
          n276 = call <vilib>:"Spark MAX Get Sensor Position.vi"("MotorControlDevRef in"=w478) -> ("Sensor Position"=w476:dbl, "MotorControlDevRef out"=w477:T3)  [unwired: 7 in, 2 out]
          n277 = Subtract(x=w476, y=16.14649681529) -> (x-y=w475:dbl)
          n278 = while {
            tunnel: w477 -> [w489]
            tunnel: [w487] -> w484
            tunnel: w479 -> [w487]
            tunnel: w475 -> [w486]
            stop <- w490 stop-if-true
            n279 = Wait (ms)(milliseconds to wait=10) -> ()  [unwired: 1 out]
            n280 = call <vilib>:"Spark MAX Get Sensor Position.vi"("MotorControlDevRef in"=w489) -> ("Sensor Position"=w491:dbl)  [unwired: 7 in, 3 out]
            n281 = Less?(x=w491, y=w486) -> (x < y?=w490:bool)
          }
          n282 = call <vilib>:"WPI_RobotDriveTankDrive.vi"("Right axis value"=w483, "Left axis value"=w483, "RobotDriveDevRef"=w484) -> ()  [unwired: 6 in, 3 out]
        }
        frame #7 {
          n283 = Wait (ms)(milliseconds to wait=100) -> ()  [unwired: 1 out]
        }
        frame #8 {
          w501 = 0.0
          n284 = Unbundle By Name(w497) -> ("Motors[]"=w502:T3[])
          n285 = call <vilib>:"WPI_RobotDriveTankDrive.vi"("Right axis value"=0.6, "Left axis value"=-0.6, "RobotDriveDevRef"=w497) -> ("RobotDriveDevRef"=w496:T8)  [unwired: 6 in, 2 out]
          n286 = Index Array(array=w502) -> (element=w504:T3)  [unwired: 1 in]
          n287 = call <vilib>:"Spark MAX Get Sensor Position.vi"("MotorControlDevRef in"=w504) -> ("Sensor Position"=w495:dbl, "MotorControlDevRef out"=w503:T3)  [unwired: 7 in, 2 out]
          n288 = Subtract(x=w495, y=15.11598261637) -> (x-y=w493:dbl)
          n289 = while {
            tunnel: w503 -> [w508]
            tunnel: [w506] -> w500
            tunnel: w496 -> [w506]
            tunnel: w493 -> [w505]
            stop <- w509 stop-if-true
            n290 = Wait (ms)(milliseconds to wait=10) -> ()  [unwired: 1 out]
            n291 = call <vilib>:"Spark MAX Get Sensor Position.vi"("MotorControlDevRef in"=w508) -> ("Sensor Position"=w510:dbl)  [unwired: 7 in, 3 out]
            n292 = Less?(x=w510, y=w505) -> (x < y?=w509:bool)
          }
          n293 = call <vilib>:"WPI_RobotDriveTankDrive.vi"("Right axis value"=w501, "Left axis value"=w501, "RobotDriveDevRef"=w500) -> ()  [unwired: 6 in, 3 out]
        }
        frame #9 {
          n294 = Wait (ms)(milliseconds to wait=100) -> ()  [unwired: 1 out]
        }
        frame #10 {
          w520 = 0.0
          n295 = Unbundle By Name(w514) -> ("Motors[]"=w521:T3[])
          n296 = Index Array(array=w521) -> (element=w523:T3)  [unwired: 1 in]
          n297 = call <vilib>:"WPI_RobotDriveTankDrive.vi"("Right axis value"=0.6, "Left axis value"=0.6, "RobotDriveDevRef"=w514) -> ("RobotDriveDevRef"=w513:T8)  [unwired: 6 in, 2 out]
          n298 = call <vilib>:"Spark MAX Get Sensor Position.vi"("MotorControlDevRef in"=w523) -> ("Sensor Position"=w518:dbl, "MotorControlDevRef out"=w522:T3)  [unwired: 7 in, 2 out]
          n299 = Add(x=w518, y=84.32059447983 ("Position")) -> (x+y=w512:dbl)
          n300 = while {
            tunnel: w522 -> [w527]
            tunnel: [w525] -> w519
            tunnel: w513 -> [w525]
            tunnel: w512 -> [w524]
            stop <- w528 stop-if-true
            n301 = Wait (ms)(milliseconds to wait=10) -> ()  [unwired: 1 out]
            n302 = call <vilib>:"Spark MAX Get Sensor Position.vi"("MotorControlDevRef in"=w527) -> ("Sensor Position"=w529:dbl)  [unwired: 7 in, 3 out]
            n303 = Greater?(x=w529, y=w524) -> (0:w528:bool)
          }
          n304 = call <vilib>:"WPI_RobotDriveTankDrive.vi"("Right axis value"=w520, "Left axis value"=w520, "RobotDriveDevRef"=w519) -> ()  [unwired: 6 in, 3 out]
        }
        frame #11 {
          n305 = Wait (ms)(milliseconds to wait=100) -> ()  [unwired: 1 out]
        }
        frame #12 {
          w539 = 0.0
          n306 = Unbundle By Name(w531) -> ("Motors[]"=w540:T3[])
          n307 = Index Array(array=w540) -> (element=w542:T3)  [unwired: 1 in]
          n308 = call <vilib>:"WPI_RobotDriveTankDrive.vi"("Right axis value"=-0.6, "Left axis value"=0.6, "RobotDriveDevRef"=w531) -> ("RobotDriveDevRef"=w532:T8)  [unwired: 6 in, 2 out]
          n309 = call <vilib>:"Spark MAX Get Sensor Position.vi"("MotorControlDevRef in"=w542) -> ("Sensor Position"=w537:dbl, "MotorControlDevRef out"=w541:T3)  [unwired: 7 in, 2 out]
          n310 = Add(x=w537, y=7.5579913 ("Position")) -> (x+y=w535:dbl)
          n311 = while {
            tunnel: w541 -> [w546]
            tunnel: [w543] -> w538
            tunnel: w535 -> [w544]
            tunnel: w532 -> [w543]
            stop <- w547 stop-if-true
            n312 = Wait (ms)(milliseconds to wait=10) -> ()  [unwired: 1 out]
            n313 = call <vilib>:"Spark MAX Get Sensor Position.vi"("MotorControlDevRef in"=w546) -> ("Sensor Position"=w548:dbl)  [unwired: 7 in, 3 out]
            n314 = Less?(x=w548, y=w544) -> (x < y?=w547:bool)
          }
          n315 = call <vilib>:"WPI_RobotDriveTankDrive.vi"("Right axis value"=w539, "Left axis value"=w539, "RobotDriveDevRef"=w538) -> ()  [unwired: 6 in, 3 out]
        }
      }
      n316 = call <vilib>:"WPI_RobotDriveRefNum Registry Get.vi"("refnum name"="Drive") -> ("RobotDriveDevRef"=w412:T8)  [unwired: 9 in, 1 out]
      n317 = call <vilib>:"WPI_MotorControlRefNum Registry Get.vi"("refnum name"="Arm") -> ("MotorControlDevRef"=w410:T3)  [unwired: 9 in, 1 out]
      n318 = call <vilib>:"WPI_RobotDriveRefNum Registry Get.vi"("refnum name"="Drive") -> ("RobotDriveDevRef"=w422:T8)  [unwired: 9 in, 1 out]
      n319 = call <vilib>:"WPI_RobotDriveRefNum Registry Get.vi"("refnum name"="Drive") -> ("RobotDriveDevRef"=w420:T8)  [unwired: 9 in, 1 out]
      n320 = call <vilib>:"WPI_RobotDriveRefNum Registry Get.vi"("refnum name"="Drive") -> ("RobotDriveDevRef"=w418:T8)  [unwired: 9 in, 1 out]
      n321 = call <vilib>:"WPI_RobotDriveRefNum Registry Get.vi"("refnum name"="Drive") -> ("RobotDriveDevRef"=w416:T8)  [unwired: 9 in, 1 out]
    }
  }
